vi "Initialize subWorkers.vi"(8 "error in":errorcluster, 11 "Base Hardware":refnum<class "Base Hardware.lvclass">) -> (0 "error out":errorcluster, 3 "dup Base Hardware out":refnum<class "Base Hardware.lvclass">)   [LabVIEW 2023, in "Abstract Hardware.lvlib" / "Base Hardware.lvclass"]
uses:
  Base Hardware.lvclass
  <vilib>/addons/_Workers/Library/Classes/Worker/Worker.lvclass
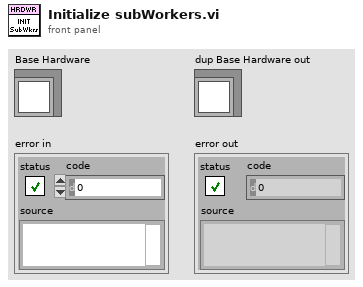
[diagram p1: front panel]
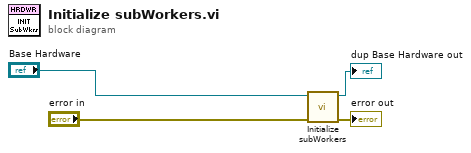
[diagram p0: block diagram]
diagram:
  n1 = call-parent "Initialize subWorkers.vi"("error in"="error in", "Worker"="Base Hardware") -> ("error out"=→"error out":errorcluster, "dup Worker out"=→"dup Base Hardware out":refnum<class "Base Hardware.lvclass">)  [unwired: 8 in]
